vi "Select Acquisition Directory for Write.vi"(0 "Autostart?":bool, 5 "Acquisition directory root path":path=path "c:/scratch", 7 "Number of acquisition files":i32) -> (4 "Sequence files handle":T1, 6 "OK?":bool)   [LabVIEW 2011]
uses:
  Sequence files handle.ctt
  GLIMPSE Globals.vi
panel:
  in  "stop":bool
  in  "Digitize to new directory":path=path "d:/1.glimpse"
  in  "Over-write exisitng:":path=path "d:/1.glimpse"
  in  "Dummy refnum array":refnum<file>[](array[refnum])
  in  "Go? (F)":bool
  in  "Over-write":bool=TRUE
  in  "New":bool
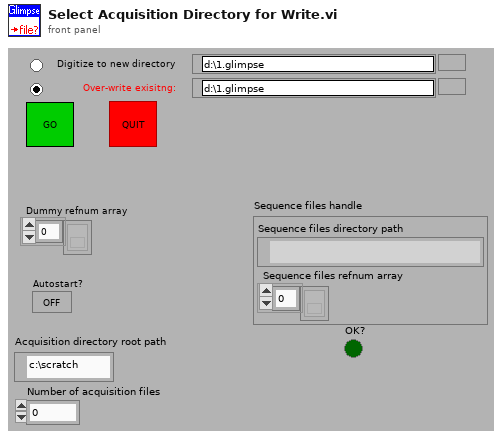
[diagram p1: front panel]
types:
  T1 = typedef "Sequence files handle.ctt" = cluster{"Sequence files directory path":path, "Sequence files refnum array":refnum<file>[]}
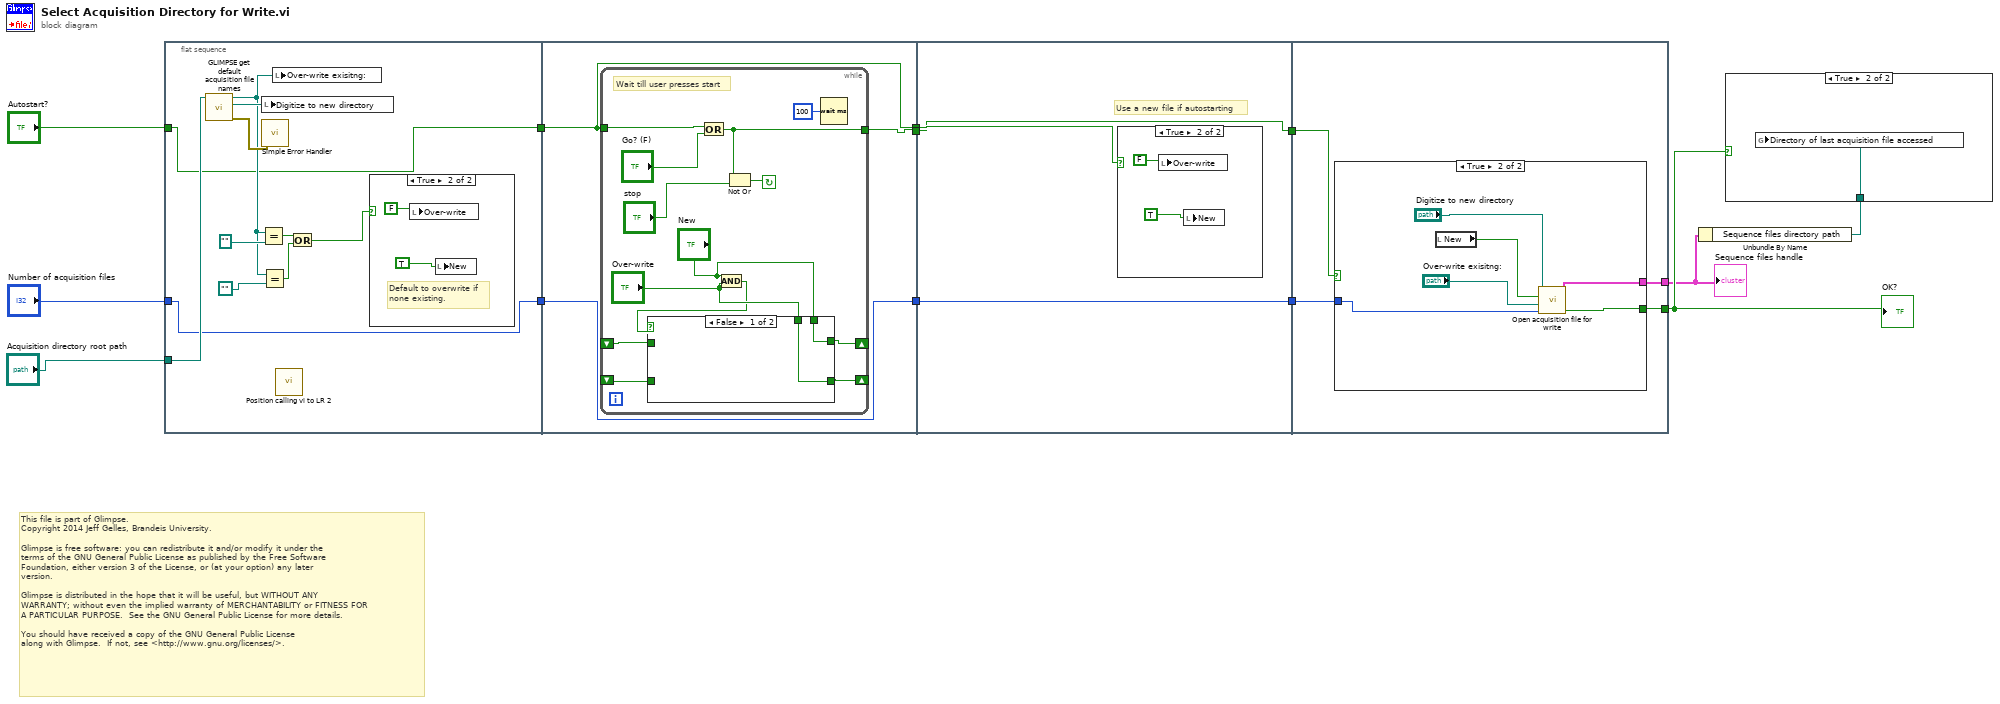
[diagram p0: block diagram]
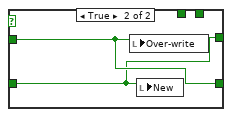
[diagram p3: hidden frame]
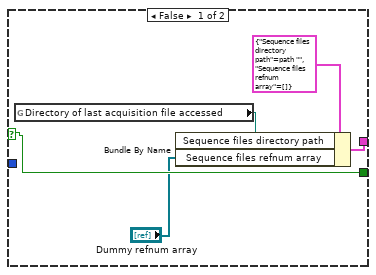
[diagram p5: hidden frame]
diagram:
  # "This file is part of Glimpse. \nCopyright 2014 Jeff Gelles, Brandeis University.    \n\nGlimpse is free software: you can redistribute it and/or modify it under the \nterms of the GNU General Public License as published by the Free Software \nFoundation, either version 3 of the License, or (at your option) any later \nversion.\n\nGlimpse is distributed in the hope that it will be useful, but WITHOUT ANY \nWARRANTY; without even the implied warranty of MERCHANTABILITY or FITNESS FOR \nA PARTICULAR PURPOSE.  See the GNU General Public License for more details.\n\nYou should have received a copy of the GNU General Public License\nalong with Glimpse.  If not, see <http://www.gnu.org/licenses/>."
  n1 = flat-sequence {
    tunnel: "Acquisition directory root path" -> [w22]
    tunnel: "Autostart?" -> [w15]
    tunnel: [w15] -> w9
    tunnel: "Number of acquisition files" -> [w14]
    tunnel: [w14] -> w8
    tunnel: w9 -> [w28]
    tunnel: [w28] -> w7
    tunnel: w8 -> [w27]
    tunnel: [w27] -> w6
    tunnel: [w29] -> w5
    tunnel: w7 -> [w49]
    tunnel: w6 -> [w48]
    tunnel: [w48] -> w4
    tunnel: w5 -> [w47]
    tunnel: [w47] -> w3
    tunnel: [w54] -> w10
    tunnel: w4 -> [w53]
    tunnel: w3 -> [w55]
    tunnel: [w52] -> w2
    frame #0 {
      n2 = call "GLIMPSE get default acquisition file names.vi"("RAID root path"=w22) -> ("error out"=w24:errorcluster, "next directory path"=w23:path, "last directory path"=w16:path)  [unwired: 1 in, 5 out]
      n3 = Equal?(x=w16, y=path "") -> (x = y?=w21:bool)
      n4 = Equal?(x=w16, y=path "") -> (x = y?=w19:bool)
      n5 = local write "Digitize to new directory"(w23) -> ()
      n6 = call <vilib>:"Simple Error Handler.vi"("error in (no error)"=w24) -> ()  [unwired: 1 in, 8 out]
      n7 = local write "Over-write exisitng:"(w16) -> ()
      n8 = call "Position calling vi to LR 2.vi"() -> ()  [unwired: 2 in, 4 out]
      n9 = Or(x=w21, y=w19) -> (x .or. y?=w20:bool)
      n10 = case shown="True" w20 {
        frame False {
        }
        frame True {
          # "Default to overwrite if\nnone existing."
          n11 = local write "Over-write"(FALSE) -> ()
          n12 = local write "New"(TRUE) -> ()
        }
      }
    }
    frame #1 {
      n13 = while {
        tunnel: [w39] -> w29
        shift-right: [w32] -> _
        shift-left: _ -> [w35]
        shift-right: [w33] -> _
        shift-left: _ -> [w34]
        tunnel: w28 -> [w31]
        stop <- w42 continue-if-true
        # "Wait till user presses start"
        n14 = Or(x=w31, y="Go? (F)") -> (x .or. y?=w39:bool)
        n15 = And(x="New", y="Over-write") -> (x .and. y?=w36:bool)
        n16 = case shown="False" w36 {
          tunnel: [w44 w45] -> w32
          tunnel: "New" -> [w44 _]
          tunnel: "Over-write" -> [w43 _]
          tunnel: [w43 w46] -> w33
          tunnel: w35 -> [_ w46]
          tunnel: w34 -> [_ w45]
          frame False {
          }
          frame True {
            n17 = local write "Over-write"(w46) -> ()
            n18 = local write "New"(w45) -> ()
          }
        }
        n19 = Not Or(1:"stop", 2:w39) -> (0:w42:bool)
        n20 = Wait (ms)(milliseconds to wait=u32 100) -> ()  [unwired: 1 out]
      }
    }
    frame #2 {
      # "Use a new file if autostarting"
      n21 = case shown="True" w49 {
        frame False {
        }
        frame True {
          n22 = local write "Over-write"(FALSE) -> ()
          n23 = local write "New"(TRUE) -> ()
        }
      }
    }
    frame #3 {
      n24 = case shown="True" w55 {
        selector: w55 -> [w60 _]
        tunnel: [w60 w65] -> w54
        tunnel: w53 -> [_ w62]
        tunnel: [w59 w61] -> w52
        frame False {
          n25 = global read "GLIMPSE Globals.vi" "Directory of last acquisition file accessed"() -> (w57:path)
          n26 = Bundle By Name(cluster=T1 {"Sequence files directory path"=path "", "Sequence files refnum array"=[]} ("Sequence files handle"), "Sequence files directory path"=w57, "Sequence files refnum array"="Dummy refnum array") -> (w59:T1)
        }
        frame True {
          n27 = local read "New"() -> (w66:bool)
          n28 = call "Open acquisition file for write.vi"("Number of acquisition files"=w62, "Existing directory to over-write"="Over-write exisitng:", "Use new?"=w66, "New directory to create"="Digitize to new directory") -> ("OK?"=w65:bool, "Sequence files handle"=w61:T1)  [unwired: 5 out]
        }
      }
    }
  }
  n29 = Unbundle By Name(w2) -> ("Sequence files directory path"=w1:path)
  n30 = case shown="True" w10 {
    tunnel: w1 -> [_ w67]
    frame False {
    }
    frame True {
      n31 = global write "GLIMPSE Globals.vi" "Directory of last acquisition file accessed"(w67) -> ()
    }
  }
  "OK?" <- w10
  "Sequence files handle" <- w2
